vi "Read Section Data.vi"(7 "Section Name":string, 8 "error in (no error)":errorcluster, 11 "Config Data":T1(array[cluster])) -> (0 "error out":errorcluster, 1 "Section Data":string[][](array[string]), 2 "Section Names":string[](array[string]), 3 "Config Data out":T1(array[cluster]), 4 "Section Exist":bool)   [LabVIEW 2020, in "GUCalibration2.lvlib"]
uses:
  GUCalibration2.lvlib
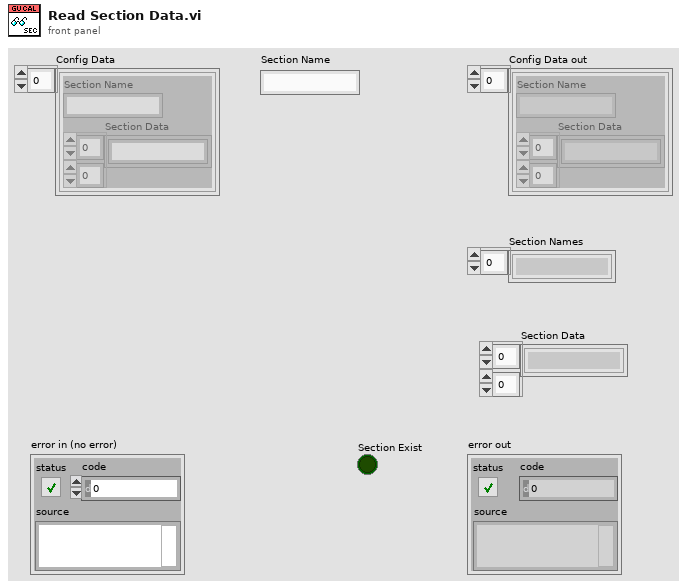
[diagram p1: front panel]
types:
  T1 = cluster{"Section Name":string, "Section Data":string[][]}[]
  T2 = cluster{"Section Name":string, "Section Data":string[][]}
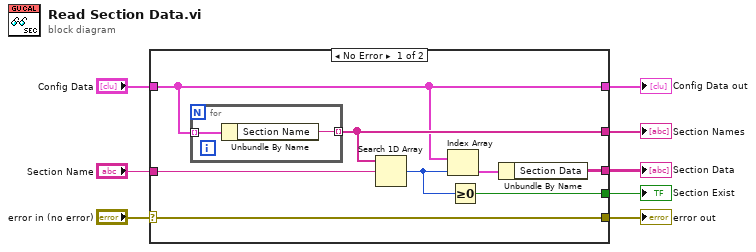
[diagram p0: block diagram]
diagram:
  n1 = case shown="No Error" "error in (no error)" {
    selector: "error in (no error)" -> [w14 w20]
    tunnel: [w16 _] -> w8
    tunnel: "Section Name" -> [w15 _]
    tunnel: "Config Data" -> [w13 w19]
    tunnel: [w14 w20] -> w4
    tunnel: [w13 w19] -> w3
    tunnel: [w11 _] -> w2
    tunnel: [w9 _] -> w1
    frame No Error {
      n2 = for {
        tunnel: w13 -> [w18] mode=indexing
        tunnel: [w17] -> w16 mode=indexing
        n3 = Unbundle By Name(w18) -> ("Section Name"=w17:string)
      }
      n4 = Search 1D Array(1D array=w16, element=w15) -> (index of element=w10:i32)  [unwired: 1 in]
      n5 = Index Array(array=w13, index=w10) -> (element=w12:T2)
      n6 = Greater Or Equal To 0?(x=w10) -> (x >= 0?=w9:bool)
      n7 = Unbundle By Name(w12) -> ("Section Data"=w11:string[][])
    }
    frame Error {
    }
  }
  "error out" <- w4
  "Section Names" <- w8
  "Config Data out" <- w3
  "Section Data" <- w2
  "Section Exist" <- w1
